vi "RemoveDC.vi"(8 "error in (no error)":errorcluster, 11 "waveform":waveform(dbl)) -> (0 "error out":errorcluster, 3 "waveform":waveform(dbl))   [LabVIEW 2017, in "EmsaAudio.lvlib"]
uses:
  <vilib>/addons/InsightCM/Devices/Shared/Emsa/EmsaAudio/EmsaAudio.lvlib
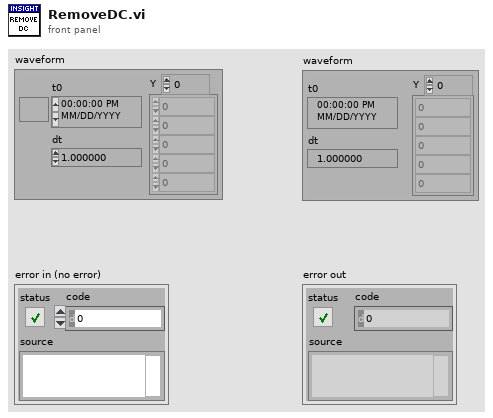
[diagram p1: front panel]
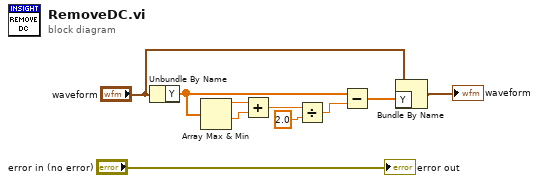
[diagram p0: block diagram]
diagram:
  n1 = Unbundle By Name("waveform") -> ("Y"=w4:dbl[])
  n2 = Array Max & Min(array=w4) -> (max value=w9:dbl, min value=w8:dbl)  [unwired: 2 out]
  n3 = Add(x=w9, y=w8) -> (x+y=w7:dbl)
  n4 = Divide(x=w7, y=2.0) -> (x/y=w5:dbl)
  n5 = Subtract(x=w4, y=w5) -> (x-y=w3:dbl[])
  n6 = Bundle By Name(cluster="waveform", "Y"=w3) -> (→"waveform":waveform(dbl))
  "error out" <- "error in (no error)"
